vi "Main.vi"() -> ()   [LabVIEW 2018]
doc: "This template is for the Queued Message Handler design pattern.\n\nThe Event Handling Loop generates messages based on user interface actions.\n\nThe Message Handling Loop processes messages generated by the Event Handling Loop, or by other messages. The messages are string values, so new messages can be added easily to the Message Cases case structure in the Message Handling Loop. Each message cluster can also provide an optional value for Message Data, which is a variant that can be converted to whatever message-specific data is required."
uses:
  controls/UI Data.ctl
  classes/Counter/Counter.lvclass
  support/Message Queue/Enqueue Message (Single).vi
  <vilib>/Utility/error.llb/Error Cluster From Error Code.vi
  <vilib>/ErrorRing/Error Ring.xnode
  support/Message Queue/Message Queue.lvlib
  support/User Event - Stop/User Event - Stop.lvlib
panel:
  in  "Reset":bool
  in  "Increment":bool
  in  "Decrement":bool
  out "Count":dbl
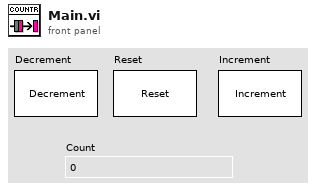
[diagram p1: front panel]
types:
  T1 = typedef "UI Data.ctl" = cluster{"Counter":refnum<class "Counter.lvclass">}
  T2 = typedef "Message Queue.lvlib/All Message Queues.ctl" = cluster{"UI":refnum<queue>}
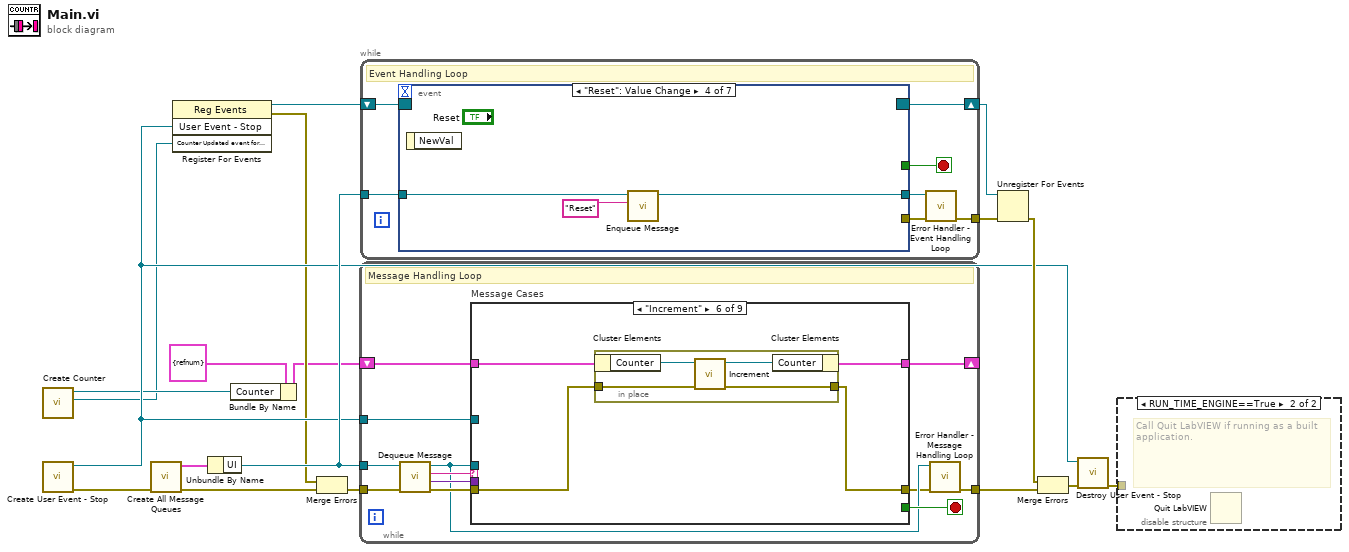
[diagram p0: block diagram]
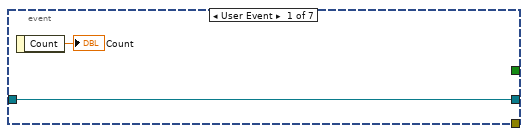
[diagram p2: hidden frame]
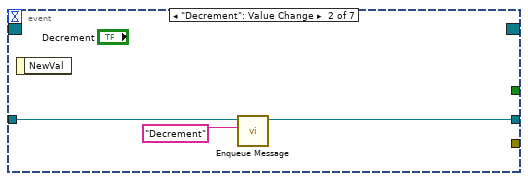
[diagram p3: hidden frame]
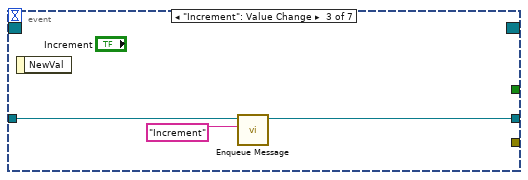
[diagram p4: hidden frame]
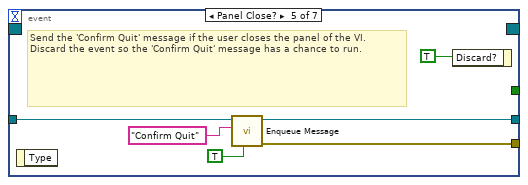
[diagram p5: hidden frame]
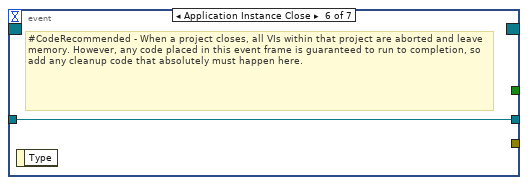
[diagram p6: hidden frame]
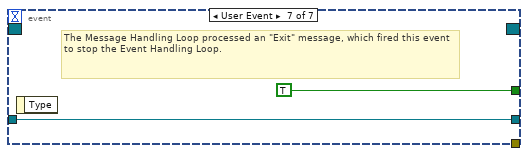
[diagram p7: hidden frame]
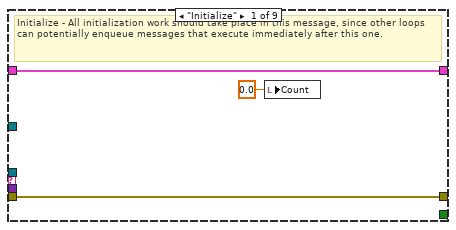
[diagram p8: hidden frame]
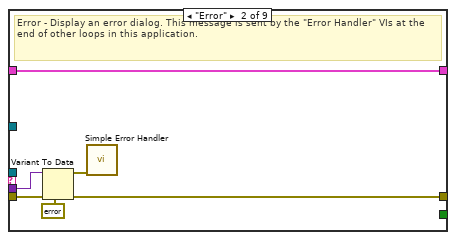
[diagram p9: hidden frame]
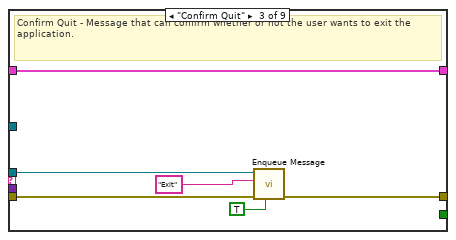
[diagram p10: hidden frame]
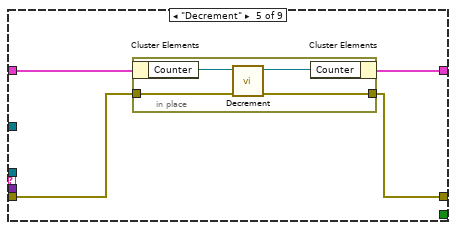
[diagram p12: hidden frame]
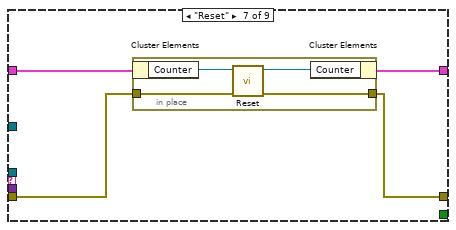
[diagram p13: hidden frame]
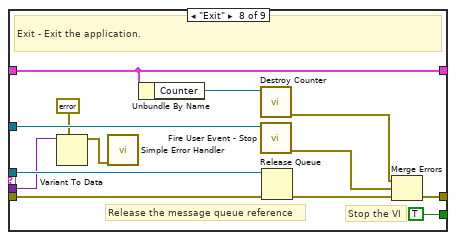
[diagram p14: hidden frame]
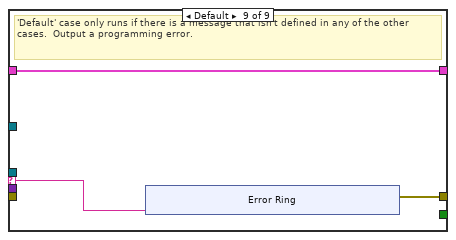
[diagram p15: hidden frame]
diagram:
  n1 = call "Create Counter.vi"() -> ("Counter Updated event for registration"=w1:refnum<user-event>, "Counter out"=w2:refnum<class "Counter.lvclass">)  [unwired: 9 in, 1 out]
  n2 = call "Create User Event - Stop.vi"() -> ("error out"=w14:errorcluster, "User Event - Stop"=w6:refnum<user-event>)  [unwired: 10 in]
  n3 = call "Create All Message Queues.vi"("error in (no error)"=w14) -> ("error out"=w18:errorcluster, "Message Queues out"=w17:T2)  [unwired: 9 in]
  n4 = register-events(w6, w1) -> (reference out=w7:refnum<event-registration>, error out=w4:errorcluster)  [unwired: 2 in]
  n5 = Unbundle By Name(w17) -> ("UI"=w15:refnum<queue>)
  n6 = Bundle By Name(cluster=T1 {"Counter"=refnum} ("Data Cluster"), "Counter"=w2) -> (w3:T1)
  n7 = Merge Errors(w4, w18) -> (w5:errorcluster)
  n8 = while {
    tunnel: w15 -> [w22]
    shift-right: [w29] -> _
    shift-left: w3 -> [w30]
    tunnel: w6 -> [w27]
    tunnel: w5 -> [w26]
    tunnel: [w20] -> w16
    stop <- w28 stop-if-true
    # "Message Handling Loop"
    n9 = call "Dequeue Message.vi"("error in (no error)"=w26, "Message Queue"=w22) -> ("error out"=w25:errorcluster, "Message Data"=w23:variant, "Message"=w24:string, "dup Message Queue"=w21:refnum<queue>)  [unwired: 6 in]
    n10 = case "Message Cases" shown="\"Increment\"" w24 {
      selector: w24 -> [_ _ _ _ _ _ _ _ w85]
      tunnel: w21 -> [_ _ w42 _ _ _ _ w84 _]
      tunnel: w25 -> [w33 w39 w45 w47 w49 w57 w65 w78 _]
      tunnel: [w33 w34 w43 w47 w48 w56 w64 w81 w86] -> w19
      tunnel: w30 -> [w32 w38 w44 w46 w51 w59 w67 w74 w87]
      tunnel: [w32 w38 w44 w46 w50 w58 w66 w74 w87] -> w29
      tunnel: [_ _ _ _ _ _ _ TRUE _] -> w28
      tunnel: w23 -> [_ w37 _ _ _ _ _ w75 _]
      tunnel: w27 -> [_ _ _ _ _ _ _ w80 _]
      frame "Initialize" {
        # "Initialize - All initialization work should take place in this message, since other loops can potentially enqueue messages that execute immediately after this one."
        n11 = local write "Count"(0.0 ("Count")) -> ()
      }
      frame "Error" {
        # "Error - Display an error dialog. This message is sent by the \"Error Handler\" VIs at the end of other loops in this application."
        n12 = Variant To Data(error in=w39, type=errorcluster {"status"=FALSE, "code"=0, "source"=""} ("error constant"), Variant=w37) -> (data=w35:errorcluster, error out=w34:errorcluster)
        n13 = call <vilib>:"Simple Error Handler.vi"("error in (no error)"=w35) -> ()  [unwired: 4 in, 5 out]
      }
      frame "Confirm Quit" {
        # "Confirm Quit - Message that can confirm whether or not the user wants to exit the application."
        n14 = call-poly "Enqueue Message.vi"("Priority Message? (F)"=TRUE, "error in (no error)"=w45, "Message"="Exit", "Message Queue"=w42) -> ("error out"=w43:errorcluster)  [unwired: 6 in, 1 out]
      }
      frame "---Copy This Frame---" {
        # "Duplicate this frame when creating new messages.  Change this comment in the duplicated frame to describe this message."
      }
      frame "Decrement" {
        n15 = in-place {
          in-place-border: w49 -> [w53]
          in-place-border: [w52] -> w48
          n16 = in-place-cluster #1(w51) -> ("Counter"=w55:refnum<class "Counter.lvclass">)
          n17 = call-dynamic "Decrement.vi"("error in (no error)"=w53, "Counter in"=w55) -> ("error out"=w52:errorcluster, "Counter out"=w54:refnum<class "Counter.lvclass">)  [unwired: 8 in]
          n18 = in-place-cluster #1("Counter"=w54) -> (w50:T1)
        }
      }
      frame "Increment" {
        n19 = in-place {
          in-place-border: w57 -> [w61]
          in-place-border: [w60] -> w56
          n20 = in-place-cluster #2(w59) -> ("Counter"=w63:refnum<class "Counter.lvclass">)
          n21 = call-dynamic "Increment.vi"("error in (no error)"=w61, "Counter in"=w63) -> ("error out"=w60:errorcluster, "Counter out"=w62:refnum<class "Counter.lvclass">)  [unwired: 8 in]
          n22 = in-place-cluster #2("Counter"=w62) -> (w58:T1)
        }
      }
      frame "Reset" {
        n23 = in-place {
          in-place-border: w65 -> [w69]
          in-place-border: [w68] -> w64
          n24 = in-place-cluster #3(w67) -> ("Counter"=w71:refnum<class "Counter.lvclass">)
          n25 = call-dynamic "Reset.vi"("error in (no error)"=w69, "Counter in"=w71) -> ("error out"=w68:errorcluster, "Counter out"=w70:refnum<class "Counter.lvclass">)  [unwired: 8 in]
          n26 = in-place-cluster #3("Counter"=w70) -> (w66:T1)
        }
      }
      frame "Exit" {
        # "Stop the VI"
        # "Release the message queue reference"
        # "Exit - Exit the application."
        n27 = Variant To Data(type=errorcluster {"status"=FALSE, "code"=0, "source"=""} ("error constant"), Variant=w75) -> (data=w76:errorcluster)  [unwired: 1 in, 1 out]
        n28 = call <vilib>:"Simple Error Handler.vi"("error in (no error)"=w76) -> ()  [unwired: 4 in, 5 out]
        n29 = Unbundle By Name(w74) -> ("Counter"=w73:refnum<class "Counter.lvclass">)
        n30 = call "Destroy Counter.vi"("Counter in"=w73) -> ("error out"=w72:errorcluster)  [unwired: 9 in, 1 out]
        n31 = call "Fire User Event - Stop.vi"("User Event - Stop"=w80) -> ("error out"=w79:errorcluster)  [unwired: 10 in]
        n32 = Release Queue(queue=w84, error in (no error)=w78) -> (error out=w82:errorcluster)  [unwired: 1 in, 2 out]
        n33 = Merge Errors(w72, w79, w82) -> (w81:errorcluster)
      }
      frame Default {
        # "'Default' case only runs if there is a message that isn't defined in any of the other cases.  Output a programming error."
        n34 = xnode "Error Ring"("parameter 0"=w85) -> ("error out"=w86:errorcluster)
      }
    }
    n35 = call "Error Handler - Message Handling Loop.vi"("error in (no error)"=w19, "Message Queue"=w21) -> ("dup error in"=w20:errorcluster)  [unwired: 8 in, 1 out]
  }
  n36 = while {
    tunnel: w15 -> [w101]
    shift-right: [w99] -> w11
    shift-left: w7 -> [w100]
    tunnel: [w95] -> w8
    stop <- w97 stop-if-true
    # "Event Handling Loop"
    n37 = event shown="[3] \"Reset\": Value Change" {
      selector: w100 -> [_ _ _ _ _ _ _]
      dyn-events: [_ _ _ _ _ _ _] -> w99
      timeout: _ -> [_ _ _ _ _ _ _]
      tunnel: [_ _ _ _ _ _ TRUE ("Discard?")] -> w97
      tunnel: w101 -> [w103 w106 w109 w112 w117 w119 w121]
      tunnel: [_ _ _ _ w116 _ _] -> w98
      tunnel: [w103 w105 w108 w111 w115 w119 w121] -> w96
      event User Event {
        n38 = event-data() -> ("Count"=→"Count":dbl)  [unwired: 1 in]
      }
      event "Decrement": Value Change {
        n39 = event-data() -> ()  [unwired: 1 in, 1 out]
        n40 = call-poly "Enqueue Message.vi"("Message"="Decrement", "Message Queue"=w106) -> ("dup Message Queue"=w105:refnum<queue>)  [unwired: 8 in, 1 out]
      }
      event "Increment": Value Change {
        n41 = event-data() -> ()  [unwired: 1 in, 1 out]
        n42 = call-poly "Enqueue Message.vi"("Message"="Increment", "Message Queue"=w109) -> ("dup Message Queue"=w108:refnum<queue>)  [unwired: 8 in, 1 out]
      }
      event "Reset": Value Change {
        n43 = event-data() -> ()  [unwired: 1 in, 1 out]
        n44 = call-poly "Enqueue Message.vi"("Message"="Reset", "Message Queue"=w112) -> ("dup Message Queue"=w111:refnum<queue>)  [unwired: 8 in, 1 out]
      }
      event Panel Close? {
        # "Send the 'Confirm Quit' message if the user closes the panel of the VI. Discard the event so the 'Confirm Quit' message has a chance to run."
        n45 = event-data() -> ()  [unwired: 1 in, 1 out]
        n46 = call-poly "Enqueue Message.vi"("Priority Message? (F)"=TRUE, "Message"="Confirm Quit", "Message Queue"=w117) -> ("error out"=w116:errorcluster, "dup Message Queue"=w115:refnum<queue>)  [unwired: 7 in]
        n47 = event-data("Discard?"=TRUE) -> ()  [unwired: 1 in, 1 out]
      }
      event Application Instance Close {
        # "#CodeRecommended - When a project closes, all VIs within that project are aborted and leave memory. However, any code placed in this event frame is guaranteed to run to completion, so add any cleanup code that absolutely must happen here."
        n48 = event-data() -> ()  [unwired: 1 in, 1 out]
      }
      event User Event {
        # "The Message Handling Loop processed an \"Exit\" message, which fired this event to stop the Event Handling Loop."
        n49 = event-data() -> ()  [unwired: 1 in, 1 out]
      }
    }
    n50 = call "Error Handler - Event Handling Loop.vi"("error in (no error)"=w98, "Message Queue"=w96) -> ("dup error in"=w95:errorcluster)  [unwired: 8 in, 1 out]
  }
  n51 = Unregister For Events(event registration refnum=w11, error in=w8) -> (error out=w12:errorcluster)
  n52 = Merge Errors(w12, w16) -> (w13:errorcluster)
  n53 = call "Destroy User Event - Stop.vi"("error in (no error)"=w13, "User Event - Stop"=w6) -> ("error out"=w9:errorcluster)  [unwired: 9 in]
  n54 = disable-structure shown="RUN_TIME_ENGINE==True" {
    disable-tunnel: w9 -> [_ _]
    frame condition #0 (active) {
    }
    frame condition #1 {
      # "Call Quit LabVIEW if running as a built application."
      n55 = Quit LabVIEW() -> ()  [unwired: 1 in]
    }
  }
